vi "spec_set_subcupconfig.vi"(8 "error in (no error)":errorcluster, 10 "subcupconfig name":string, 11 "Qtegra in":refnum<class "Qtegra.lvclass">) -> (0 "error out":errorcluster, 2 "value out":string, 3 "Qtegra out":refnum<class "Qtegra.lvclass">)   [LabVIEW 2017, in "Qtegra.lvclass"]
doc: "sets the supcupconfiguration of the selected instrument object. The subcupconfiguration is give as the name of the config.\nThis mainly applies to QTegra\n\nIt is not checked whether the subcupconfiguartion actually exists on the instrument"
uses:
  Qtegra.lvclass
  \\Mac\Home/my data/University/Lamont/Software/LabView/MSControlSuite_Code/MSControl/Classes/Instrument/instrument.lvclass
  global variables.vi
  instrument.lvclass
  StatusLog/StatusLog.lvclass
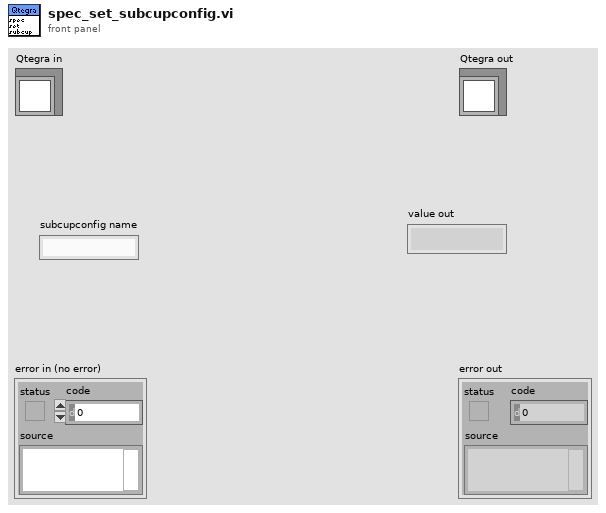
[diagram p1: front panel]
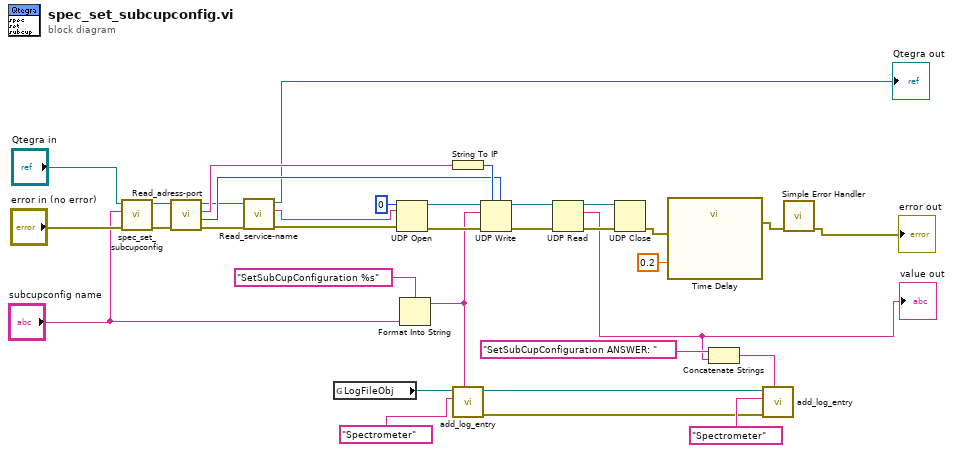
[diagram p0: block diagram]
diagram:
  n1 = call-parent "spec_set_subcupconfig.vi"("error in (no error)"="error in (no error)", "subcupconfig name"="subcupconfig name", "instrument in"="Qtegra in") -> ("error out"=w4:errorcluster, "instrument out"=w5:refnum<class "Qtegra.lvclass">)  [unwired: 6 in, 1 out]
  n2 = call "Read_adress-port.vi"("error in (no error)"=w4, "instrument in"=w5) -> ("error out"=w24:errorcluster, "port number"=w25:i32, "adress"=w32:string, "instrument out"=w23:refnum<class "Qtegra.lvclass">)  [unwired: 6 in]
  n3 = call-dynamic "Read_service-name.vi"("error in (no error)"=w24, "instrument in"=w23) -> ("error out"=w22:errorcluster, "service name"=w21:string, "instrument out"=→"Qtegra out":refnum<class "Qtegra.lvclass">)  [unwired: 7 in]
  n4 = global read "global variables.vi" "LogFileObj"() -> (w11:refnum<class "StatusLog.lvclass">)
  n5 = UDP Open(8:w22, 10:w21, 11:u16 0 ("port")) -> (port=w28:refnum<k16>, 0:w29:errorcluster)  [unwired: 2 in, 1 out]
  n6 = Format Into String(format string="SetSubCupConfiguration %s", "subcupconfig name") -> (resulting string=w13:string)  [unwired: 2 in, 1 out]
  n7 = String To IP(1:w32) -> (0:w31:u32)
  n8 = call-dynamic "add_log_entry.vi"("new entry"=w13, "log identifiers"="Spectrometer", "StatusLog in"=w11) -> ("error out"=w7:errorcluster, "StatusLog out"=w10:refnum<class "StatusLog.lvclass">)  [unwired: 5 in]
  n9 = UDP Write(address=w31, port or service name=w25, connection ID=w28, data in=w13, 8:w29) -> (error out=w26:errorcluster, 3:w27:refnum<k16>)  [unwired: 1 in]
  n10 = UDP Read(connection ID=w27, 8:w26) -> (data out=w1:string, error out=w19:errorcluster, 3:w18:refnum<k16>)  [unwired: 2 in, 2 out]
  "value out" <- w1
  n11 = UDP Close(connection ID=w18, 8:w19) -> (error out=w17:errorcluster)  [unwired: 1 out]
  n12 = call "Time Delay"("error in (no error)"=w17, "Delay Time (s)"=0.2) -> ("error out"=w16:errorcluster)  [unwired: 9 in]
  n13 = Concatenate Strings("SetSubCupConfiguration ANSWER: ", w1) -> (w8:string)
  n14 = call-dynamic "add_log_entry.vi"("new entry"=w8, "error in (no error)"=w7, "log identifiers"="Spectrometer", "StatusLog in"=w10) -> ()  [unwired: 4 in, 2 out]
  n15 = call <vilib>:"Simple Error Handler.vi"("error in (no error)"=w16) -> ("error out"=→"error out":errorcluster)  [unwired: 4 in, 4 out]
